vi "ByteArray_OpenMV.vi"(11 "String":string) -> (0 "slash codes ignored":u8[](array[numeric]) format="%.0x", 1 "Array":u8[](array[numeric]), 3 "string":string)   [LabVIEW 2022 SP3]
panel:
  out "string 3":string
  out "string 2":string
  out "Numeric":u8 format="%.0x"
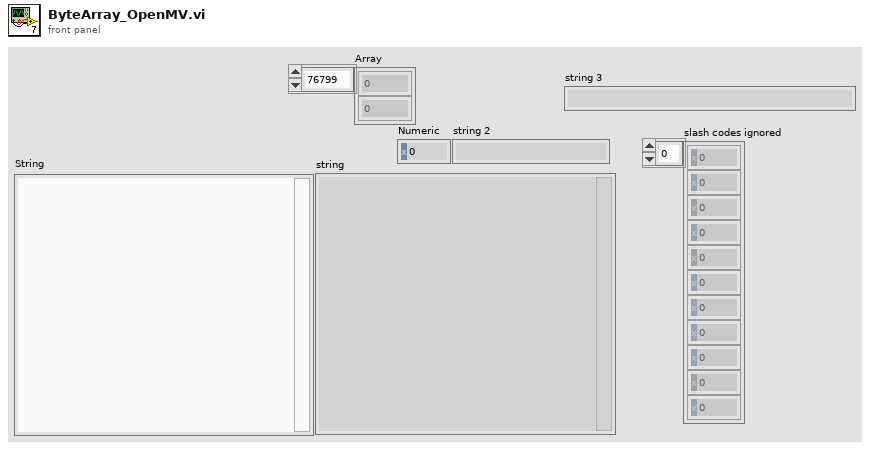
[diagram p1: front panel]
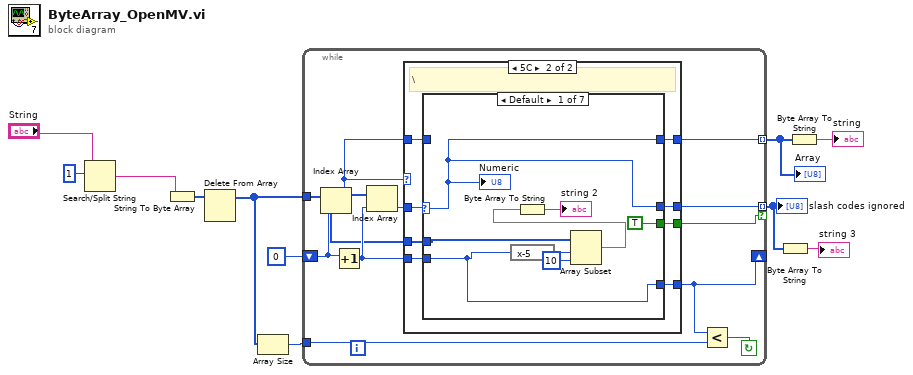
[diagram p0: block diagram]
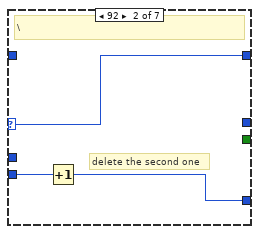
[diagram p3: hidden frame]
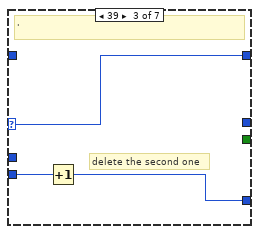
[diagram p4: hidden frame]
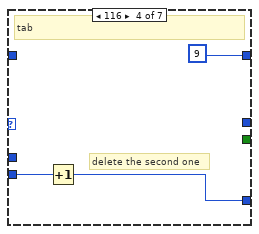
[diagram p5: hidden frame]
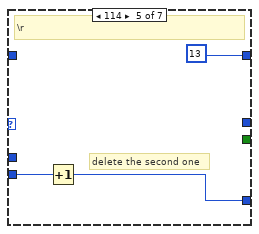
[diagram p6: hidden frame]
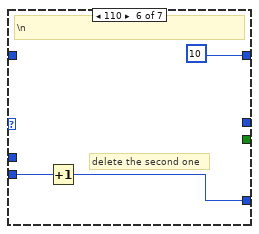
[diagram p7: hidden frame]
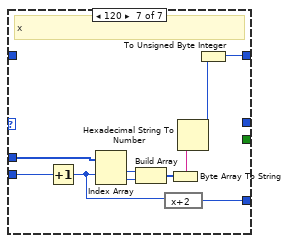
[diagram p8: hidden frame]
diagram:
  n1 = Search/Split String(string="String", offset (0)=1) -> (match + rest of string=w3:string)  [unwired: 1 in, 2 out]
  n2 = String To Byte Array(string=w3) -> (unsigned byte array=w2:u8[])
  n3 = Delete From Array(array=w2) -> (array with subset deleted=w1:u8[])  [unwired: 2 in, 1 out]
  n4 = Array Size(array=w1) -> (size(s)=w8:i32)
  n5 = while {
    tunnel: w1 -> [w19]
    shift-right: [w18] -> _
    shift-left: u32 0 -> [w22]
    tunnel: [w21] -> w10 mode=indexing
    tunnel: w8 -> [w17]
    tunnel: [w13] -> w6 mode=indexing if=w12
    stop <- w16 continue-if-true
    n6 = Index Array(array=w19, index=w22) -> (element=w15:u8)
    n7 = Increment(x=w22) -> (x+1=w20:u32)
    n8 = Index Array(array=w19, index=w20) -> (element=w14:u8)
    n9 = case shown="5C" w15 {
      tunnel: w20 -> [w24 w32]
      tunnel: [w24 w31] -> w18
      tunnel: w19 -> [_ w30]
      tunnel: [w23 w29] -> w21
      tunnel: w15 -> [w23 w27]
      tunnel: w14 -> [_ w28]
      tunnel: [_ w26] -> w13
      tunnel: [_ w25] -> w12
      frame 0, Default {
      }
      frame 92 {
        # "\\"
        n10 = case shown="Default" w28 {
          selector: w28 -> [w35 w42 w45 _ _ _ _]
          tunnel: w32 -> [w33 w43 w46 w49 w52 w55 w65]
          tunnel: [w33 w41 w44 w48 w51 w54 w64] -> w31
          tunnel: w30 -> [w39 _ _ _ _ _ w61]
          tunnel: [w35 w42 w45 u8 9 u8 13 u8 10 w57] -> w29
          tunnel: w27 -> [_ _ _ _ _ _ _]
          tunnel: [w35 _ _ _ _ _ _] -> w26
          tunnel: [TRUE _ _ _ _ _ _] -> w25
          frame Default {
            n11 = expression code="x-5"(w33) -> (w36:u32)
            n12 = Array Subset(array=w39, index=w36, length=10) -> (w37:u8[])
            n13 = Byte Array To String(unsigned byte array=w37) -> (string=→"string 2":string)
            "Numeric" <- w35
          }
          frame 92 {
            # "delete the second one"
            # "\\"
            n14 = Increment(x=w43) -> (x+1=w41:u32)
          }
          frame 39 {
            # "delete the second one"
            # "'"
            n15 = Increment(x=w46) -> (x+1=w44:u32)
          }
          frame 116 {
            # "delete the second one"
            # "tab"
            n16 = Increment(x=w49) -> (x+1=w48:u32)
          }
          frame 114 {
            # "delete the second one"
            # "\\r"
            n17 = Increment(x=w52) -> (x+1=w51:u32)
          }
          frame 110 {
            # "delete the second one"
            # "\\n"
            n18 = Increment(x=w55) -> (x+1=w54:u32)
          }
          frame 120 {
            # "x"
            n19 = Increment(x=w65) -> (x+1=w56:u32)
            n20 = Index Array(array=w61, index #1=w56) -> (element #1=w62:u8, element #2=w63:u8)  [unwired: 1 in]
            n21 = Build Array(w62, w63) -> (w60:u8[])
            n22 = expression code="x+2"(w56) -> (w64:u32)
            n23 = Byte Array To String(unsigned byte array=w60) -> (string=w59:string)
            n24 = Hexadecimal String To Number(string=w59) -> (number=w58:u32)  [unwired: 2 in, 1 out]
            n25 = To Unsigned Byte Integer(number=w58) -> (unsigned 8bit integer=w57:u8)
          }
        }
      }
    }
    n26 = Less?(x=w18, y=w17) -> (x < y?=w16:bool)
  }
  "Array" <- w10
  "slash codes ignored" <- w6
  n27 = Byte Array To String(unsigned byte array=w6) -> (string=→"string 3":string)
  n28 = Byte Array To String(unsigned byte array=w10) -> (string=→"string":string)
